vi "Flatten_ClassGen.vi"(8 "error in (no error)":errorcluster caption="entrée d'erreur (pas d'erreur)", 9 "XML File Path":path, 11 "Objet LabVIEW":refnum<class>) -> (0 "error out":errorcluster caption="sortie d'erreur", 1 "XML File Path Out":path caption="Chemin du fichier XML (duplicata)", 2 "Data Class Flattened to XML String":string)   [LabVIEW 2019]
uses:
  <vilib>/Utility/xml.llb/Write to XML File(string).vi
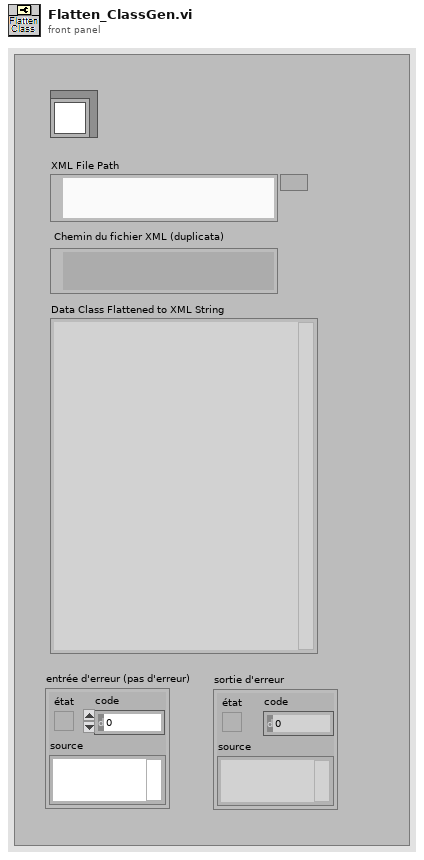
[diagram p1: front panel]
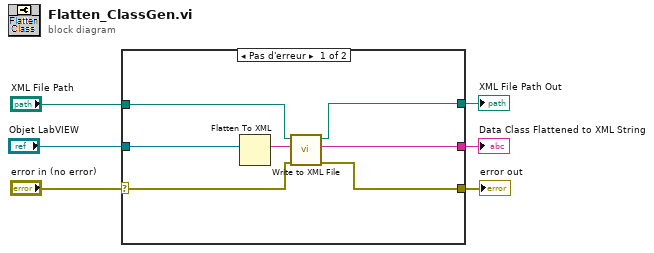
[diagram p0: block diagram]
diagram:
  n1 = case shown="Pas d'erreur" "error in (no error)" {
    selector: "error in (no error)" -> [w11 w14]
    tunnel: "Objet LabVIEW" -> [w13 _]
    tunnel: "XML File Path" -> [w10 w15]
    tunnel: [w9 w15] -> w4
    tunnel: [w8 _] -> w3
    tunnel: [w7 w14] -> w2
    frame No Error {
      n2 = Flatten To XML(anything=w13) -> (xml string=w12:string)
      n3 = call-poly <vilib>:"Write to XML File.vi"("error in (no error)"=w11, "XML Input"=w12, "XML File Path"=w10) -> ("error out"=w7:errorcluster, "XML String"=w8:string, "XML File Path(duplicate)"=w9:path)  [unwired: 6 in]
    }
    frame Error {
    }
  }
  "error out" <- w2
  "Data Class Flattened to XML String" <- w3
  "XML File Path Out" <- w4
